vi "V-Meter Configure (3706).vi"(8 "error in (no error)":errorcluster, 11 "VISA resource name in":refnum<visa-resource-name>) -> (0 "error out":errorcluster, 3 "VISA resource name out":refnum<visa-resource-name>)   [LabVIEW 2016, in "Hall Effect Library.lvlib"]
uses:
  Hall Effect Library.lvlib
  Global Variables/Test Settings.vi
  <instrlib>/Keithley 3706/Keithley 3706.lvlib
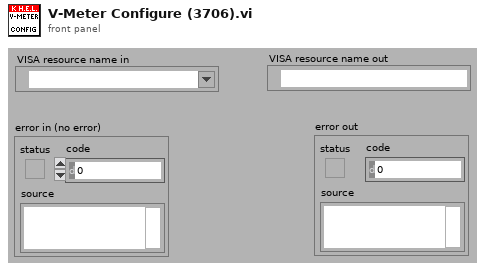
[diagram p1: front panel]
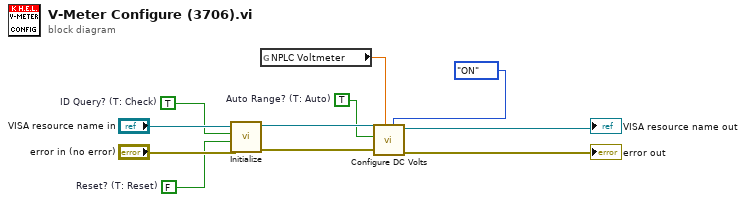
[diagram p0: block diagram]
diagram:
  w5 = TRUE  # Auto Range? (T: Auto)
  w9 = TRUE  # ID Query? (T: Check)
  w8 = FALSE  # Reset? (T: Reset)
  n1 = call <instrlib>:"Initialize.vi"("error in (no error)"="error in (no error)", "Reset (True)"=w8, "ID Query (True)"=w9, "VISA resource name"="VISA resource name in") -> ("error out"=w6:errorcluster, "VISA resource name out"=w7:refnum<visa-resource-name>)  [unwired: 6 in]
  n2 = global read "Test Settings.vi" "NPLC Voltmeter"() -> (w4:dbl)
  n3 = call <instrlib>:"Configure DC Volts.vi"("AutoZero"=enum16{"OFF", "ON", "ONCE"}."ON", "NPLC"=w4, "error in"=w6, "AutoRange  On"=w5, "VISA resource name"=w7) -> ("error out"=→"error out":errorcluster, "VISA resource name out"=→"VISA resource name out":refnum<visa-resource-name>)  [unwired: 4 in, 1 out]
